vi "Plate Configuration.vi"() -> ()   [LabVIEW 2015]
panel:
  out "출력 클러스터":T1
  in  "Internal Control Label":T2(array[cluster])=[{"Row Index"="A", "Internal Ctrl"=FALSE}, {"Row Index"="B", "Internal Ctrl"=FALSE}, {"Row Index"="C", "Internal Ctrl"=FALSE}, {"Row Index"="D", "Internal Ctrl"=FALSE}, {"Row Index"="E", "Internal Ctrl"=FALSE}, {"Row Index"="F", "Internal Ctrl"=FALSE}, {"Row Index"="G", "Internal Ctrl"=FALSE}, {"Row Index"="H", "Internal Ctrl"=TRUE}]
  in  "정지 버튼":bool
  in  "Technical replicate":i32
  in  "Experimental Group Label":cluster{string, "Group Label":bool}[](array[cluster])=[{"01", "Group Label"=FALSE}, {"02", "Group Label"=FALSE}, {"03", "Group Label"=FALSE}, {"04", "Group Label"=FALSE}, {"05", "Group Label"=FALSE}, {"06", "Group Label"=FALSE}, {"07", "Group Label"=TRUE}, {"08", "Group Label"=TRUE}, {"09", "Group Label"=TRUE}, {"10", "Group Label"=TRUE}, {"11", "Group Label"=TRUE}, {"12", "Group Label"=TRUE}]
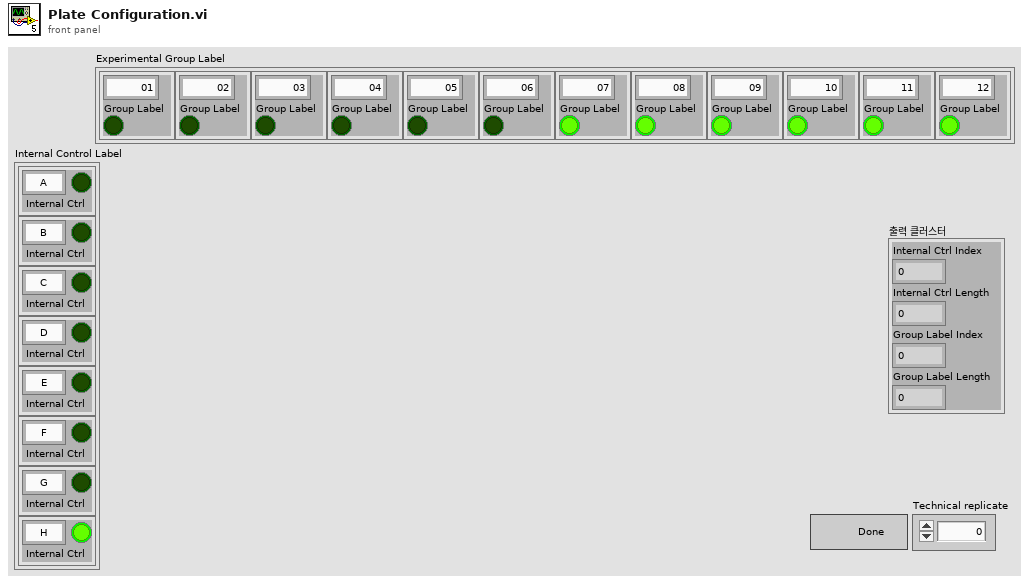
[diagram p1: front panel]
types:
  T1 = cluster{"Internal Ctrl Index":i32, "Internal Ctrl Length":i32, "Group Label Index":i32, "Group Label Length":i32}
  T2 = cluster{"Row Index":string, "Internal Ctrl":bool}[]
  T3 = cluster{"Internal Ctrl Index":i32, "Internal Ctrl Length":i32, i32, i32}
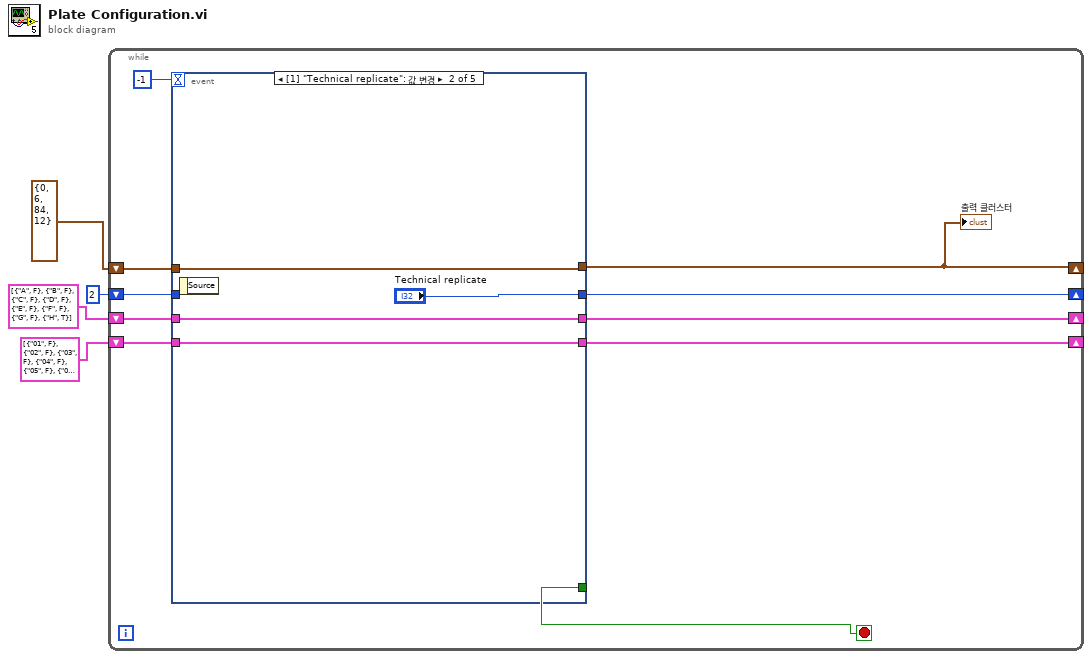
[diagram p0: block diagram]
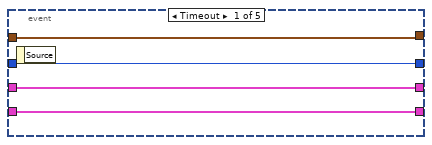
[diagram p2: hidden frame]
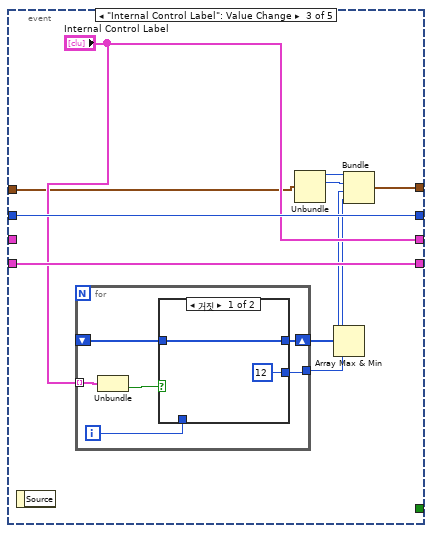
[diagram p3: hidden frame]
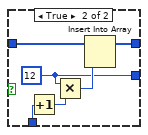
[diagram p4: hidden frame]
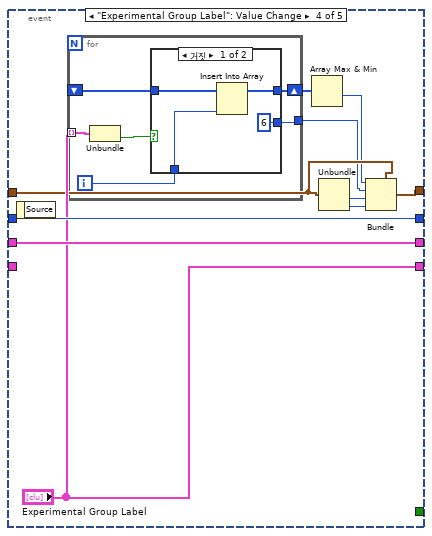
[diagram p5: hidden frame]
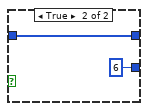
[diagram p6: hidden frame]
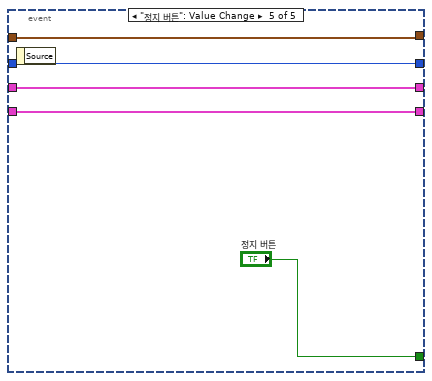
[diagram p7: hidden frame]
diagram:
  n1 = while {
    shift-right: [w12] -> _
    shift-left: 2 ("Technical replicate") -> [w11]
    shift-right: [w7] -> _
    shift-left: T2 [{"Row Index"="A", "Internal Ctrl"=FALSE}, {"Row Index"="B", "Internal Ctrl"=FALSE}, {"Row Index"="C", "Internal Ctrl"=FALSE}, {"Row Index"="D", "Internal Ctrl"=FALSE}, {"Row Index"="E", "Internal Ctrl"=FALSE}, {"Row Index"="F", "Internal Ctrl"=FALSE}, {"Row Index"="G", "Internal Ctrl"=FALSE}, {"Row Index"="H", "Internal Ctrl"=TRUE}] ("Internal Control Label 2") -> [w10]
    shift-right: [w8] -> _
    shift-left: cluster{string, "Group Label":bool}[] [{"01", "Group Label"=FALSE}, {"02", "Group Label"=FALSE}, {"03", "Group Label"=FALSE}, {"04", "Group Label"=FALSE}, {"05", "Group Label"=FALSE}, {"06", "Group Label"=FALSE}, {"07", "Group Label"=TRUE}, {"08", "Group Label"=TRUE}, {"09", "Group Label"=TRUE}, {"10", "Group Label"=TRUE}, {"11", "Group Label"=TRUE}, {"12", "Group Label"=TRUE}] ("Experimental Group Label 2") -> [w9]
    shift-right: [w5] -> _
    shift-left: T1 {"Internal Ctrl Index"=0, "Internal Ctrl Length"=6, "Group Label Index"=84, "Group Label Length"=12} ("출력 클러스터 2") -> [w6]
    stop <- w13 stop-if-true
    n2 = event shown="[1] \"Technical replicate\": 값 변경" {
      selector: _ -> [_ _ _ _ _]
      dyn-events: _ -> [_ _ _ _ _]
      timeout: -1 -> [_ _ _ _ _]
      tunnel: [_ _ _ _ "정지 버튼"] -> w13
      tunnel: [w18 "Technical replicate" w31 _ w72] -> w12
      tunnel: [w17 w21 "Internal Control Label" w55 w71] -> w7
      tunnel: [w16 w20 w32 "Experimental Group Label" w70] -> w8
      tunnel: w11 -> [w18 _ w31 w56 w72]
      tunnel: w10 -> [w17 w21 _ w55 w71]
      tunnel: w9 -> [w16 w20 w32 _ w70]
      tunnel: [_ _ _ w56 _] -> _
      tunnel: w6 -> [w15 w19 w28 w51 w69]
      tunnel: [w15 w19 w27 w52 w69] -> w5
      event Timeout {
        n3 = event-data() -> ()  [unwired: 1 in, 1 out]
      }
      event "Technical replicate": Value Change {
        n4 = event-data() -> ()  [unwired: 1 in, 1 out]
      }
      event "Internal Control Label": Value Change {
        n5 = event-data() -> ()  [unwired: 1 in, 1 out]
        n6 = for {
          tunnel: "Internal Control Label" -> [w38] mode=indexing
          shift-right: [w35] -> w29
          shift-left: _ -> [w34]
          tunnel: [w33] -> w23
          i -> [w36]
          n7 = Unbundle(w38) -> ("Internal Ctrl"=w37:bool)  [unwired: 1 out]
          n8 = case shown="거짓" w37 {
            tunnel: w36 -> [_ w43]
            tunnel: [w40 w45] -> w35
            tunnel: w34 -> [w40 w44]
            tunnel: [12 w41] -> w33
            frame False {
            }
            frame True {
              w41 = 12
              n9 = Increment(x=w43) -> (x+1=w42:i32)
              n10 = Multiply(x=w41, y=w42) -> (x*y=w46:i32)
              n11 = Insert Into Array(array=w44, new element=w46) -> (w45:i32[])  [unwired: 1 in]
            }
          }
        }
        n12 = Unbundle(w28) -> ("Internal Ctrl Index"=w26:i32, "Internal Ctrl Length"=w25:i32)  [unwired: 2 out]
        n13 = Array Max & Min(array=w29) -> (min value=w24:i32)  [unwired: 3 out]
        n14 = Bundle("Internal Ctrl Index"=w26, "Internal Ctrl Length"=w25, w24, w23) -> (w27:T3)  [unwired: 1 in]
      }
      event "Experimental Group Label": Value Change {
        n15 = event-data() -> ()  [unwired: 1 in, 1 out]
        n16 = for {
          tunnel: "Experimental Group Label" -> [w62] mode=indexing
          shift-right: [w59] -> w53
          shift-left: _ -> [w58]
          tunnel: [w57] -> w47
          i -> [w60]
          n17 = Unbundle(w62) -> ("Group Label"=w61:bool)  [unwired: 1 out]
          n18 = case shown="거짓" w61 {
            tunnel: w60 -> [w64 _]
            tunnel: [w66 w68] -> w59
            tunnel: w58 -> [w65 w68]
            tunnel: [6 6] -> w57
            frame False {
              n19 = Insert Into Array(array=w65, new element=w64) -> (w66:i32[])  [unwired: 1 in]
            }
            frame True {
            }
          }
        }
        n20 = Array Max & Min(array=w53) -> (min value=w48:i32)  [unwired: 3 out]
        n21 = Unbundle(w51) -> ("Group Label Index"=w50:i32, "Group Label Length"=w49:i32)  [unwired: 2 out]
        n22 = Bundle(cluster=w51, "Internal Ctrl Index"=w48, "Internal Ctrl Length"=w47, "Group Label Index"=w50, "Group Label Length"=w49) -> (w52:T1)
      }
      event "정지 버튼": Value Change {
        n23 = event-data() -> ()  [unwired: 1 in, 1 out]
      }
    }
    "출력 클러스터" <- w5
  }
